vi "Komponent Beschreibung Tabelle.vi"(4 "Sprachliste":string[][](array[string]), 6 "Modus":T3 caption="Modus:" items=["Messen", "CG zu Entnahmestelle"], 7 "Komponenten":T1 caption="Cluster", 9 "Max Fehler":string, 10 "Table Header":string[](array[string]), 11 "TestKonfig":T4 {"TestKonfig Interferent"."Gasflasche MFC3" items=["----"=10000, "IAG NH3 3000"=0, "IAG NH3 200"=1, "IAG NH3 2000"=2, "IAG MG"=3, "IAG O2"=4]; "TestKonfig Interferent"."Gasflasche MFC2" items=["----"=10000, "IAG NH3 3000"=0, "IAG NH3 200"=1, "IAG NH3 2000"=2, "IAG MG"=3, "IAG O2"=4]; "TestKonfig Interferent"."Eingangs Konzentration MFC1" min=0.0; "TestKonfig Interferent"."Ausgangs Konzentration MFC1" min=0.0; "TestKonfig Interferent"."MFC2" items=["MFC 2", "MFC 3", "MFC 4", "MFC 5"]; "TestKonfig Interferent"."MFC3" items=["MFC 2", "MFC 3", "MFC 4", "MFC 5"]; "TestKonfig Interferent"."Ausgangs Konzentration MFC3" min=0.0; "TestKonfig Interferent"."Eingangs Konzentration MFC3" min=0.0; "TestKonfig Interferent"."Ausgangs Konzentration MFC2" min=0.0; "TestKonfig Interferent"."Eingangs Konzentration MFC2" min=0.0; "TestKonfig H2O"."HovaCAL Temperature" format="%.2f"; "TestKonfig H2O"."HovaCAL Flow Input Cluster"."HovaCAL Flow Input Cluster" format="%.2f"; "TestKonfig H2O"."Eingangs Konzentration:" min=0.0; "TestKonfig H2O"."zusätzliche Zeitdauer Erster Punkt" min=30 step=1 format="%#_5g"; "TestKonfig H2O"."Zeitdauer Stufen" format="%#_5g"; "TestKonfig H2O"."Max Fehler" format="%#_5g"; "TestKonfig H2O"."Anzahl Stufen" format="%#_5g"; "TestKonfig H2O"."Modus" items=["Messen", "CG zu Entnahmestelle"]}) -> (3 "Tabelle":string[][](array[string]))   [LabVIEW 2020, in "EPA 1065.lvlib" / "HovaCAL Interference verificaton.lvlib"]
uses:
  HovaCAL Interference verificaton.lvlib
  TestKonfig.ctl
  TestKonfig H2O.ctl
  Modus.ctl
  Linearisierung V2/SpanEinstellungen/Einheit.ctl
  Linearisierung V2/Gasteiler/Stufen Tabelle 10 Stufen.ctl
  Linearisierung V2/Gasteiler/HovaCAL_Interface/Controls/Flow Einstellung.ctl
  Linearisierung V2/Gasteiler/HovaCAL_Interface/Controls/Temp Sollwerte Anzeige.ctl
  TestKonfig Interferents.ctl
  MFCAuswahl.ctl
  Seiten/System Einstellungen V2/Gasflasche Auswahl.ctl
  Linearisierung V2/Gasteiler/HovaCAL_Interface/Kommunikation/Aktion_FGV_HovaCAL_Interface_GetData.ctl
  Sprachverwaltung/Sprachverwaltung.lvlib
  Linearisierung V2/SpanEinstellungen/SpanEinstellungen.lvlib
  Linearisierung V2/Gasteiler/HovaCAL_Interface/Kommunikation/Kommunikation.lvlib
  Linearisierung V2/Gasteiler/HovaCAL_Interface/Controls/Controls.lvlib
  Seiten/System Einstellungen V2/System Einstellungen V2.lvlib
  Linearisierung V2/Gasteiler/Gasteiler.lvlib
  Visualisierungs Elemente/String - Ausgabefeld.ctl
  Komponenten.ctl
panel:
  # "sec"
  # "%"
  # "sec"
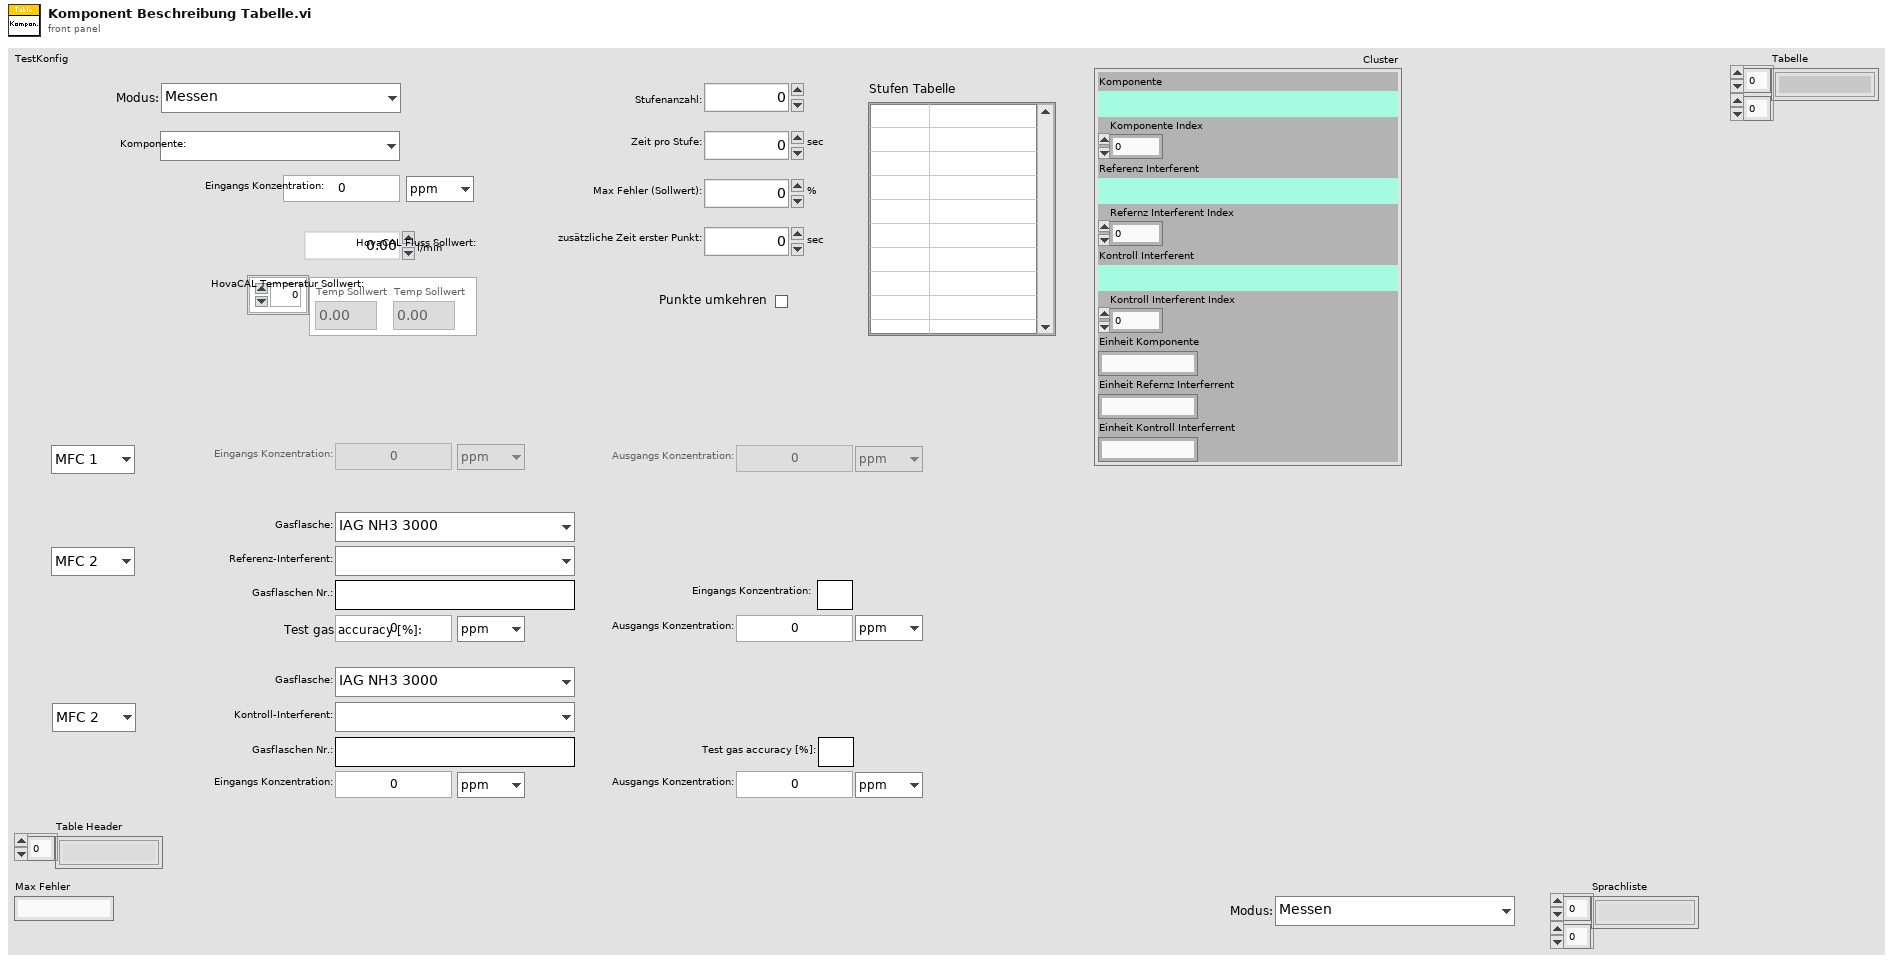
[diagram p1: front panel]
types:
  T1 = typedef "EPA 1065.lvlib/HovaCAL Interference verificaton.lvlib/Komponenten.ctl" = cluster{"Komponente":T2, "Komponente Index":i32, "Referenz Interferent":T2, "Refernz Interferent Index":i32, "Kontroll Interferent":T2, "Kontroll Interferent Index":i32, "Einheit Komponente":string, "Einheit Refernz Interferrent":string, "Einheit Kontroll Interferrent":string}
  T2 = typedef "String - Ausgabefeld.ctl" = string
  T3 = typedef "EPA 1065.lvlib/HovaCAL Interference verificaton.lvlib/Modus.ctl" = u16
  T4 = typedef "EPA 1065.lvlib/HovaCAL Interference verificaton.lvlib/TestKonfig.ctl" = cluster{"TestKonfig H2O":T5, "TestKonfig Interferent":T10}
  T5 = typedef "EPA 1065.lvlib/HovaCAL Interference verificaton.lvlib/TestKonfig H2O.ctl" = cluster{"Modus":T3, "Komponente:":u16, "Eingangs Konzentration:":dbl, "Einheit":T6, "Anzahl Stufen":sgl, "Zeitdauer Stufen":sgl, "Max Fehler":sgl, "zusätzliche Zeitdauer Erster Punkt":sgl, "Punkte umkehren":bool, "Stufen Tabelle":T7, "HovaCAL Flow Input Cluster":T8, "HovaCAL Temperature":T9}
  T6 = typedef "Linearisierung v2.lvlib/SpanEinstellungen.lvlib/Einheit.ctl" = enum16{"ppm", "%"}
  T7 = typedef "Linearisierung v2.lvlib/Gasteiler.lvlib/Stufen Tabelle 10 Stufen.ctl" = string[][]
  T8 = typedef "Linearisierung v2.lvlib/Gasteiler.lvlib/HovaCAL_Interface.lvlib/Controls.lvlib/Flow Einstellung.ctl" = cluster{"HovaCAL Flow Input Cluster":dbl}
  T9 = typedef "Linearisierung v2.lvlib/Gasteiler.lvlib/HovaCAL_Interface.lvlib/Controls.lvlib/Temp Sollwerte Anzeige.ctl" = dbl[]
  T10 = typedef "EPA 1065.lvlib/HovaCAL Interference verificaton.lvlib/TestKonfig Interferents.ctl" = cluster{"MFC1":enum16{"MFC 1"}, "Eingangs Konzentration MFC1":dbl, "Einheit MFC1 Eingang":T6, "Ausgangs Konzentration MFC1":dbl, "Einheit MFC1 Ausgang":T6, "MFC2":T11, "Referenz-Interferent:":u16, "Gasflaschen Nr MFC2":string, "Accuracy MFC2":string, "Eingangs Konzentration MFC2":dbl, "Einheit MFC2 Eingang":T6, "Ausgangs Konzentration MFC2":dbl, "Einheit MFC2 Ausgang":T6, "MFC3":T11, "Kontroll-Interferent:":u16, "Gasflaschen Nr MFC3":string, "Accuracy MFC3":string, "Eingangs Konzentration MFC3":dbl, "Einheit MFC3 Eingang":T6, "Ausgangs Konzentration MFC3":dbl, "Einheit MFC3 Ausgang":T6, "Gasflasche MFC2":T12, "Gasflasche MFC3":T12}
  T11 = typedef "EPA 1065.lvlib/HovaCAL Interference verificaton.lvlib/MFCAuswahl.ctl" = u16
  T12 = typedef "System Einstellungen V2.lvlib/Gasflasche Auswahl.ctl" = u16
  T13 = typedef "Linearisierung v2.lvlib/Gasteiler.lvlib/HovaCAL_Interface.lvlib/Kommunikation.lvlib/Aktion_FGV_HovaCAL_Interface_GetData.ctl" = enum16{"lesen", "SystemInfo", "MFC Info", "actual Values", "Limits", "first contact", "reset after read"}
  T14 = typedef "Linearisierung v2.lvlib/Gasteiler.lvlib/HovaCAL_Interface.lvlib/Controls.lvlib/Info Cluster.ctl" = cluster{"device":string, "version":string, "number of mfc":i32, "number of pumps":i32, "number of temp controllers":i32, "number of mfs":i32, "number of balances":i32}
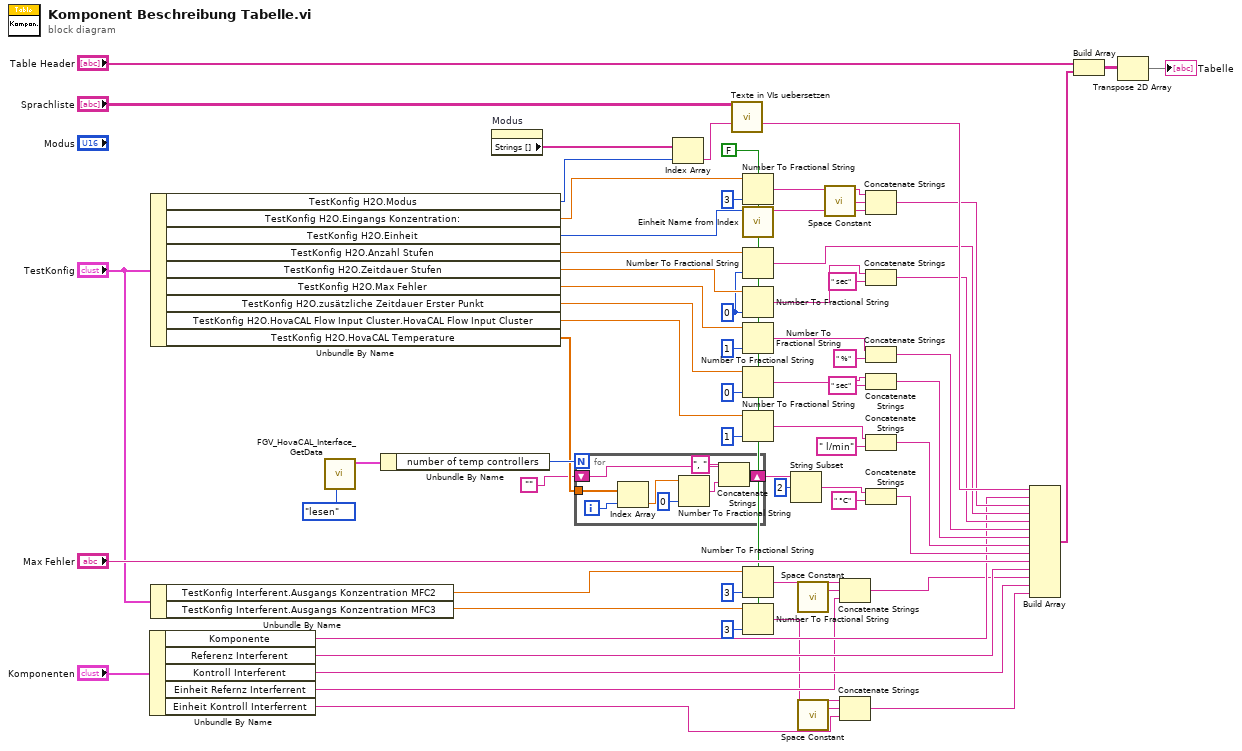
[diagram p0: block diagram]
diagram:
  w20 = i16 0 ("Genauigkeit (6)")
  w13 = FALSE ("Systemdezimalzeichen verwenden (T)")
  n1 = Unbundle By Name("Komponenten") -> ("Komponente"=w17:T2, "Referenz Interferent"=w10:T2, "Kontroll Interferent"=w9:T2, "Einheit Refernz Interferrent"=w6:string, "Einheit Kontroll Interferrent"=w2:string)
  n2 = Unbundle By Name("TestKonfig") -> ("TestKonfig H2O.Modus"=w66:T3, "TestKonfig H2O.Eingangs Konzentration:"=w58:dbl, "TestKonfig H2O.Einheit"=w56:T6, "TestKonfig H2O.Anzahl Stufen"=w21:sgl, "TestKonfig H2O.Zeitdauer Stufen"=w22:sgl, "TestKonfig H2O.Max Fehler"=w47:sgl, "TestKonfig H2O.zusätzliche Zeitdauer Erster Punkt"=w36:sgl, "TestKonfig H2O.HovaCAL Flow Input Cluster.HovaCAL Flow Input Cluster"=w35:dbl, "TestKonfig H2O.HovaCAL Temperature"=w28:T9)
  n3 = Unbundle By Name("TestKonfig") -> ("TestKonfig Interferent.Ausgangs Konzentration MFC2"=w12:dbl, "TestKonfig Interferent.Ausgangs Konzentration MFC3"=w11:dbl)
  n4 = call "FGV_HovaCAL_Interface_GetData.vi"("Aktion"=Aktion_FGV_HovaCAL_Interface_GetData."lesen") -> ("System Cluster out"=w31:T14)  [unwired: 6 in, 4 out]
  n5 = Unbundle By Name(w31) -> ("number of temp controllers"=w29:i32)
  n6 = property on="Modus" class="Ring (strikt)"() -> ("Strings []"=w67:string[])  [unwired: 2 in, 2 out]
  n7 = for {
    N: w29 -> [_]
    tunnel: w28 -> [w75]
    shift-right: [w70] -> w26
    shift-left: "" -> [w69]
    i -> [w74]
    n8 = Index Array(array=w75, index=w74) -> (element=w72:dbl)
    n9 = Number To Fractional String(number=w72, precision (6)=i16 0 ("Genauigkeit (6)")) -> (F-format string=w71:string)  [unwired: 2 in]
    n10 = Concatenate Strings(w69, ", " ("String"), w71) -> (w70:string)
  }
  n11 = Index Array(array=w67, index=w66) -> (element=w64:string)
  n12 = call "Texte in VIs uebersetzen.vi"("Sprachliste"="Sprachliste", "String zum Übersetzen"=w64) -> ("String zum Übersetzen"=w63:string)  [unwired: 9 in, 4 out]
  n13 = Number To Fractional String(use system decimal point (T)=w13, number=w58, precision (6)=i16 3 ("Genauigkeit (6)")) -> (F-format string=w53:string)  [unwired: 1 in]
  n14 = call "Einheit Name from Index.vi"("EinheitIndex"=w56) -> ("EinheitName"=w55:string)  [unwired: 10 in]
  n15 = Number To Fractional String(use system decimal point (T)=w13, number=w21, precision (6)=w20) -> (F-format string=w19:string)  [unwired: 1 in]
  n16 = Number To Fractional String(use system decimal point (T)=w13, number=w22, precision (6)=w20) -> (F-format string=w50:string)  [unwired: 1 in]
  n17 = Number To Fractional String(use system decimal point (T)=w13, number=w47, precision (6)=i16 1 ("Genauigkeit (6)")) -> (F-format string=w45:string)  [unwired: 1 in]
  n18 = Number To Fractional String(use system decimal point (T)=w13, number=w36, precision (6)=i16 0 ("Genauigkeit (6)")) -> (F-format string=w41:string)  [unwired: 1 in]
  n19 = Number To Fractional String(use system decimal point (T)=w13, number=w35, precision (6)=i16 1 ("Genauigkeit (6)")) -> (F-format string=w37:string)  [unwired: 1 in]
  n20 = Number To Fractional String(use system decimal point (T)=w13, number=w12, precision (6)=i16 3 ("Genauigkeit (6)")) -> (F-format string=w8:string)  [unwired: 1 in]
  n21 = Number To Fractional String(use system decimal point (T)=w13, number=w11, precision (6)=i16 3 ("Genauigkeit (6)")) -> (F-format string=w3:string)  [unwired: 1 in]
  n22 = String Subset(string=w26, offset (0)=2 ("Offset (0)")) -> (substring=w25:string)  [unwired: 1 in]
  n23 = call <vilib>:"Space Constant.vi"() -> ("String"=w7:string)
  n24 = call <vilib>:"Space Constant.vi"() -> ("String"=w4:string)
  n25 = call <vilib>:"Space Constant.vi"() -> ("String"=w52:string)
  n26 = Concatenate Strings(w8, w7, w6) -> (w5:string)
  n27 = Concatenate Strings(w3, w4, w2) -> (w1:string)
  n28 = Concatenate Strings(w53, w52, w55) -> (w54:string)
  n29 = Concatenate Strings(w50, " sec" ("String")) -> (w49:string)
  n30 = Concatenate Strings(w45, " %" ("String")) -> (w44:string)
  n31 = Concatenate Strings(w41, " sec" ("String")) -> (w40:string)
  n32 = Concatenate Strings(w37, " l/min" ("String")) -> (w34:string)
  n33 = Concatenate Strings(w25, " °C" ("String")) -> (w32:string)
  n34 = Build Array(w63, w17, w54, w19, w49, w44, w40, w34, w32, "Max Fehler", w10, w5, w9, w1) -> (w60:T2[])
  n35 = Build Array("Table Header", w60) -> (w59:T2[][])
  n36 = Transpose 2D Array(2D array=w59) -> (transposed array=→"Tabelle":T2[][])
